vi "Gasteiler Daten ermitteln.vi"(11 "Gasteiler":T1 caption="Analysator") -> (1 "Gasteiler Letzte Wartung":timestamp, 2 "Name für Protokoll":string, 3 "Seriennummer":string)   [LabVIEW 2020]
uses:
  Analysatoren.ctl
  Aktion FGV SystemEinstellungenV2.ctl
  System Einstellungen V2.lvlib
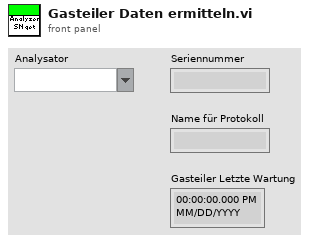
[diagram p1: front panel]
types:
  T1 = typedef "System Einstellungen V2.lvlib/Analysatoren.ctl" = string
  T2 = typedef "System Einstellungen V2.lvlib/Aktion FGV SystemEinstellungenV2.ctl" = enum16{"lesen", "Analysatoren schreiben", "Analysatoren löschen", "laden", "speichern", "Untertitel", "Analysatoren", "Neue Analysatoren", "Gasteiler schreiben", "Gasteiler löschen", "Gasteiler"}
  T3 = typedef "System Einstellungen V2.lvlib/Gasteiler.ctl" = cluster{"Gasteiler Name":string, "Gasteiler Type":string, "Gasteiler Seriennummer":string, "Gasteiler Letzte Wartung":timestamp}
  T4 = cluster{"GasteilerDefinitionsListe":T3[], "GasteilerDefinitionTextliste":string[][], "Gasteiler Strings And Values":cluster{"String":string, "Wert":string}[]}
  T5 = cluster{"Gasteiler":T1, "Gasteiler":T1, "Gasteiler":T1, "seconds since 1Jan1904":timestamp}
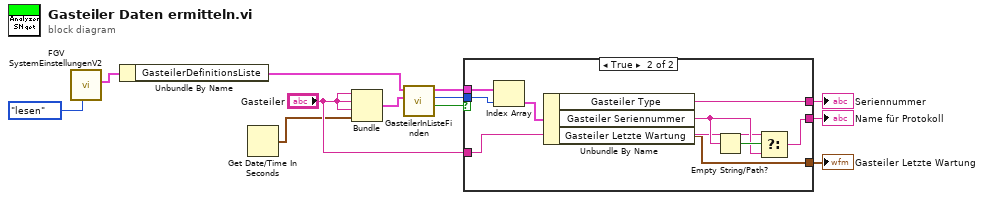
[diagram p0: block diagram]
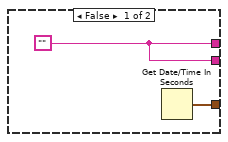
[diagram p2: hidden frame]
diagram:
  n1 = call "FGV SystemEinstellungenV2.vi"("Aktion"=Aktion_FGV_SystemEinstellungenV2."lesen") -> ("Gasteiler"=w4:T4)  [unwired: 5 in, 5 out]
  n2 = Unbundle By Name(w4) -> ("GasteilerDefinitionsListe"=w5:T3[])
  n3 = Get Date/Time In Seconds() -> (seconds since 1Jan1904=w2:timestamp)
  n4 = Bundle("Gasteiler"="Gasteiler", "Gasteiler"="Gasteiler", "Gasteiler"="Gasteiler", "seconds since 1Jan1904"=w2) -> (w3:T5)  [unwired: 1 in]
  n5 = call "GasteilerInListeFinden.vi"("Gasteiler definition"=w3, "GasteilerListe"=w5) -> ("gefunden"=w9:bool, "Index"=w10:i32, "GasteilerListe out"=w8:T3[])  [unwired: 7 in]
  n6 = case shown="True" w9 {
    tunnel: w8 -> [_ w22]
    tunnel: w10 -> [_ w21]
    tunnel: [w14 w20] -> w12
    tunnel: [w14 w16] -> w7
    tunnel: "Gasteiler" -> [_ w17]
    tunnel: [w13 w15] -> w1
    frame False {
      w14 = ""
      n7 = Get Date/Time In Seconds() -> (seconds since 1Jan1904=w13:timestamp)
    }
    frame True {
      n8 = Index Array(array=w22, index=w21) -> (element=w23:T3)
      n9 = Unbundle By Name(w23) -> ("Gasteiler Type"=w20:string, "Gasteiler Seriennummer"=w18:string, "Gasteiler Letzte Wartung"=w15:timestamp)
      n10 = Empty String/Path?(string/path=w18) -> (empty?=w19:bool)
      n11 = Select(t=w17, s=w19, f=w18) -> (s? t:f=w16:T1)
    }
  }
  "Seriennummer" <- w12
  "Name für Protokoll" <- w7
  "Gasteiler Letzte Wartung" <- w1
